vi "Autonomous Independent.vi"   [LabVIEW 2019]
doc: "This VI is called when autonomous begins, and will automatically be terminated when autonomous ends. You can carry out timed or sensor driven robot movement independently without needing to return to the caller."
uses:
  <vilib>/Rock Robotics/WPI/DriverStation/WPI_DriverStationDerivedRobotMode.ctl
  <vilib>/Rock Robotics/Network Tables/NT Read String.vi
  <vilib>/Rock Robotics/WPI/Utilities/WPI_GetSetVariantRefNum.vi
  <vilib>/Rock Robotics/Network Tables/NT Write Boolean.vi
  <vilib>/Rock Robotics/Network Tables/NT Write Number.vi
  <vilib>/Rock Robotics/Network Tables/NT Read Number.vi
  Robot Global Data.vi
  <vilib>/Rock Robotics/Network Tables/NT Write Numeric Array.vi
panel:
  # "Be sure to right-click and choose Data Operations>>Make Current Value default if you want to save the array values with the VI"
types:
  T1 = typedef "WPI_JoystickDevRef.ctl" = cluster{"Device":T2}
  T2 = typedef "WPI_JoystickDeviceEnum.ctl" = enum16{"USB 0", "USB 1", "USB 2", "USB 3", "USB 4", "USB 5"}
  T3 = typedef "WPI_MotorControlDeviceRef.ctl" = cluster{"DeviceStatus":errorcluster, "Type":T4, "PWM":cluster{"PWM Channel":T5, "DeadBand":T6}, "CAN":cluster{"Device Number":u8, "SetOutput VI Ref":variant, "GetOutput VI Ref":variant, "Enable VI Ref":variant, "Disable VI Ref":variant, "Data":variant}, "Invert":bool, "DIO PWM":cluster{"PWM \"Enable\" Channel":T5, "DIOChannel":T7, "PWM Rate":dbl}}
  T4 = typedef "WPI_MotorControlType.ctl" = enum16{"PWM", "CAN", "DIO PWM"}
  T5 = typedef "FPGA_DIOPWMChannel.ctl" = enum8{"PWM 0", "PWM 1", "PWM 2", "PWM 3", "PWM 4", "PWM 5", "PWM 6", "PWM 7", "PWM 8", "PWM 9", "PWM MXP 0", "PWM MXP 1", "PWM MXP 2", "PWM MXP 3", "PWM MXP 4", "PWM MXP 5", "PWM MXP 6", "PWM MXP 7", "PWM MXP 8", "PWM MXP 9", "Invalid"}
  T6 = typedef "WPI_PWMDeadband.ctl" = cluster{"Name":string, "maxPositivePwm":i32, "minPositivePwm":i32, "centerPwm":i32, "maxNegativePwm":i32, "minNegativePwm":i32, "angularRange":u16}
  T7 = typedef "FPGA_DIOChannel.ctl" = enum8{"DIO 0", "DIO 1", "DIO 2", "DIO 3", "DIO 4", "DIO 5", "DIO 6", "DIO 7", "DIO 8", "DIO 9", "DIO MXP 0", "DIO MXP 1", "DIO MXP 2", "DIO MXP 3", "DIO MXP 4", "DIO MXP 5", "DIO MXP 6", "DIO MXP 7", "DIO MXP 8", "DIO MXP 9", "DIO MXP 10", "DIO MXP 11", "DIO MXP 12", "DIO MXP 13", "DIO MXP 14", "DIO MXP 15", "SPI Port CS1", "SPI Port CS2", "SPI Port CS3", "SPI Port MISO", "SPI Port MOSI", "Invalid"}
  T8 = typedef "WPI_RobotDriveDevRef.ctl" = cluster{"DevStatus":errorcluster, "Motors[]":T3[], "Square Inputs":bool, "Max Output":dbl}
  T9 = typedef "WPI_DriverStationDerivedRobotMode.ctl" = enum16{"Init", "Execute", "Stop"}
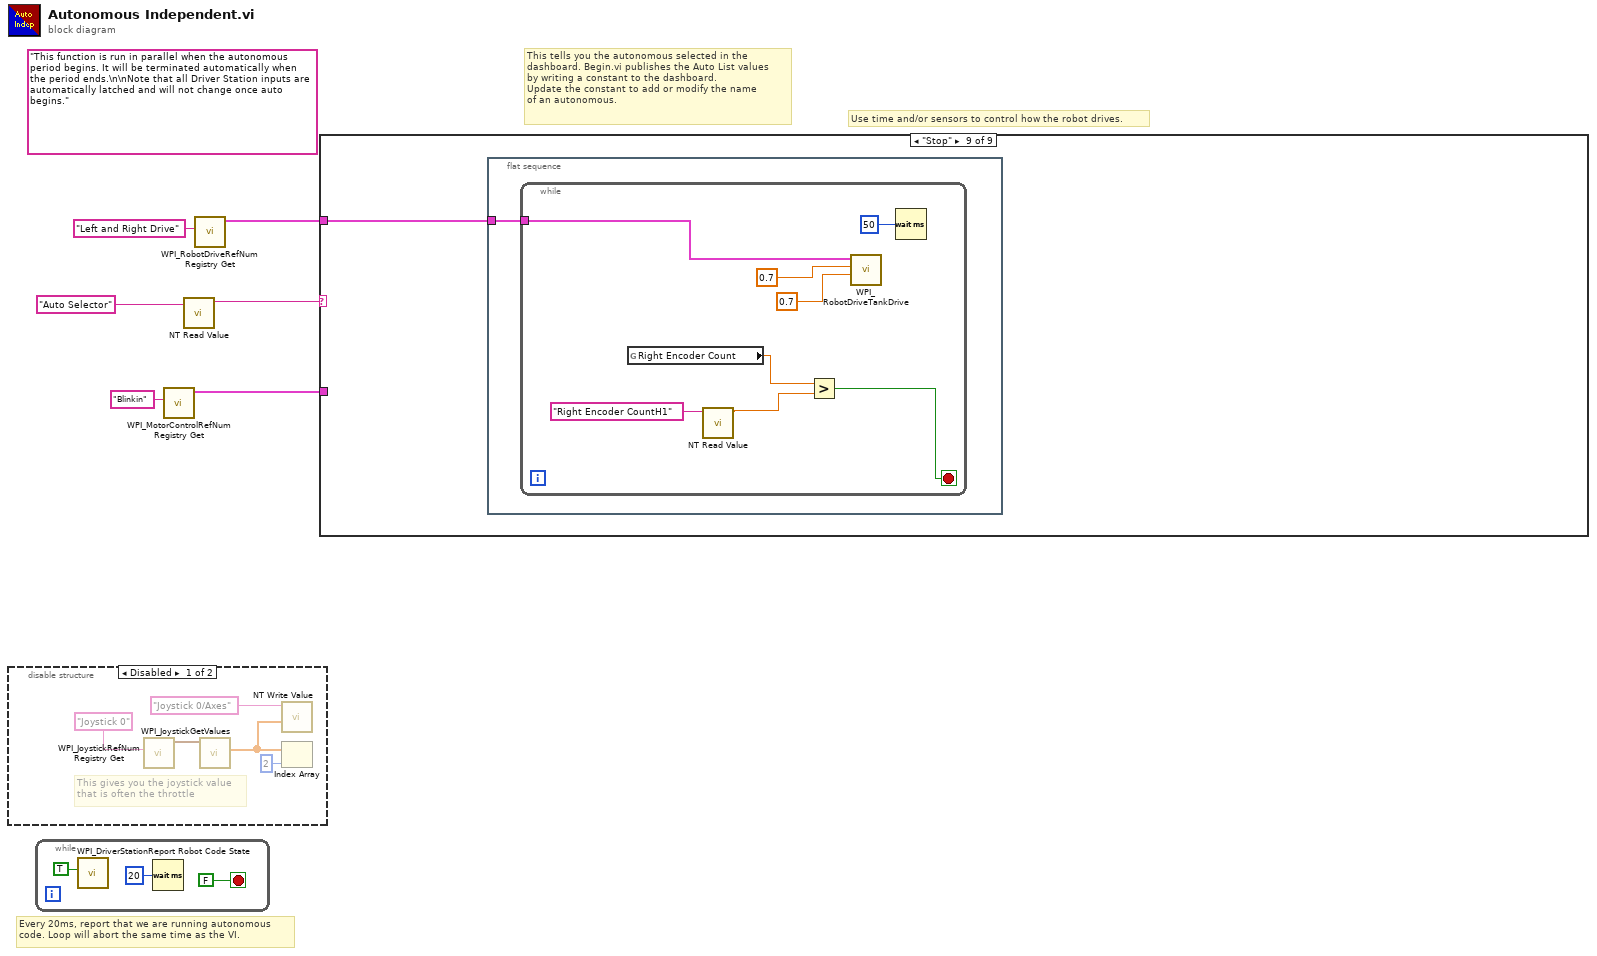
[diagram p0: block diagram]
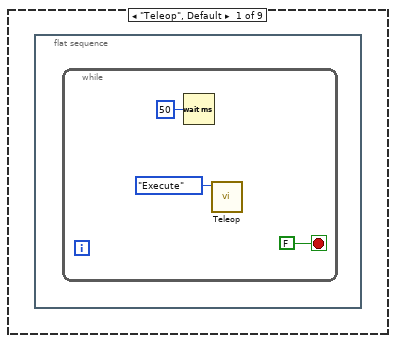
[diagram p3: hidden frame]
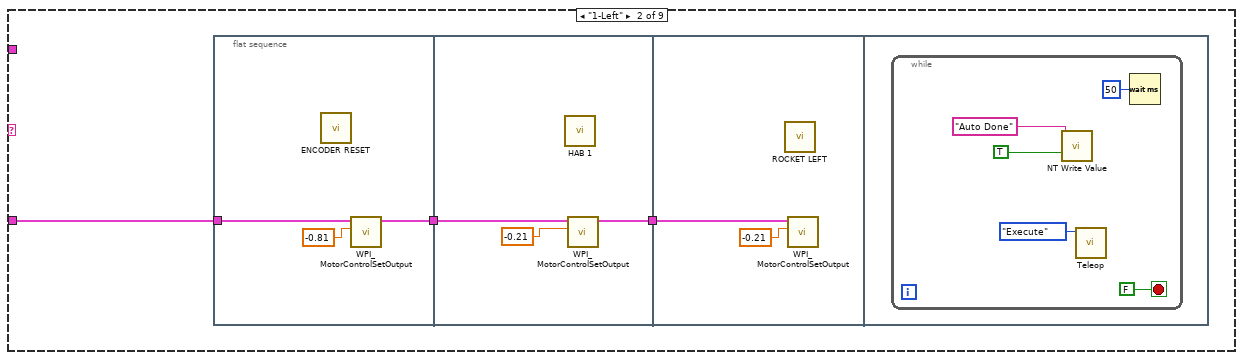
[diagram p4: hidden frame]
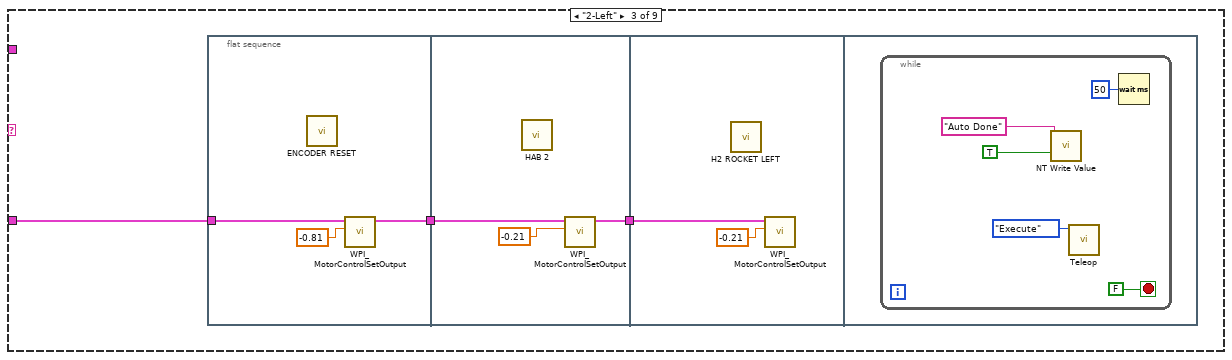
[diagram p5: hidden frame]
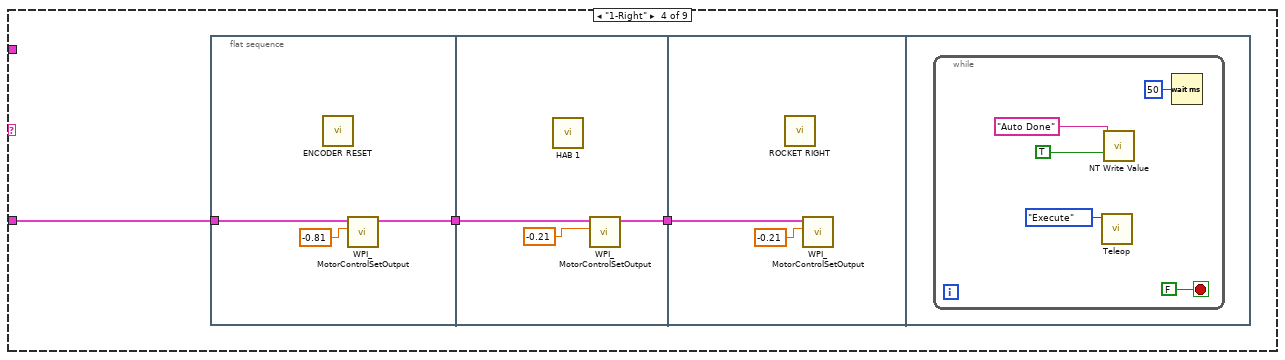
[diagram p6: hidden frame]
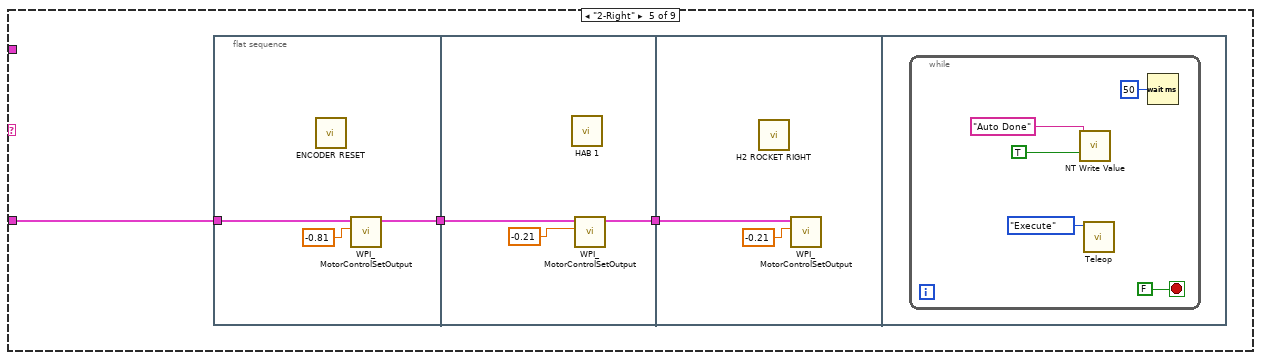
[diagram p7: hidden frame]
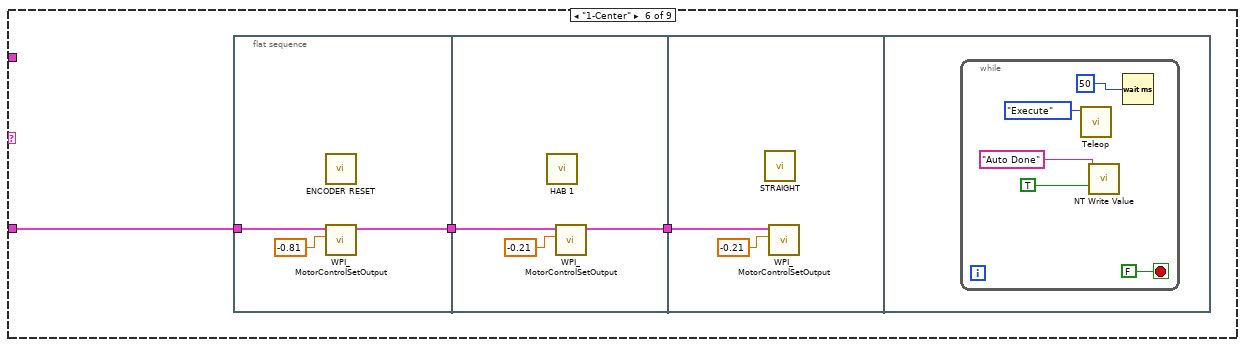
[diagram p8: hidden frame]
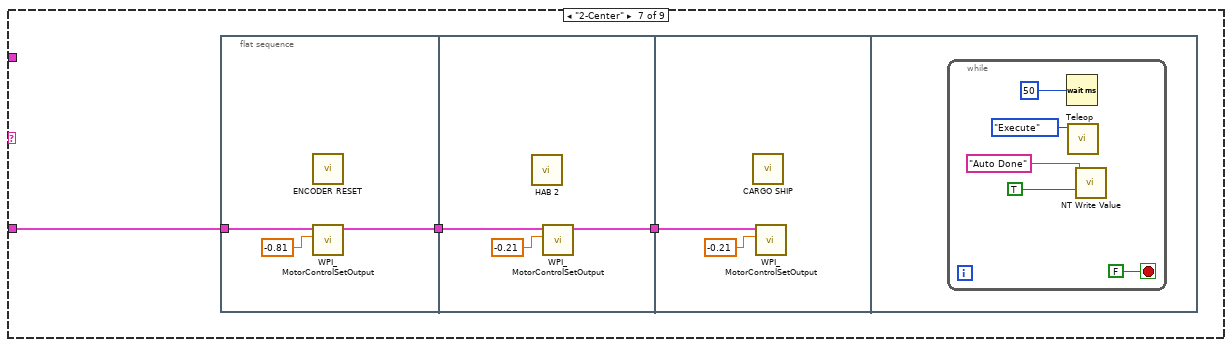
[diagram p9: hidden frame]
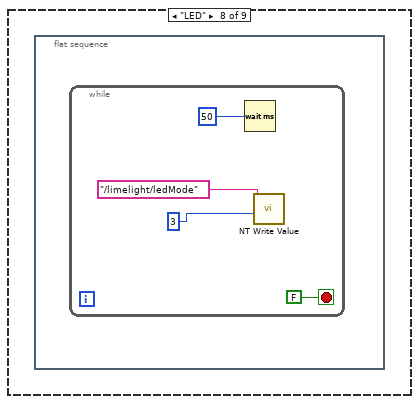
[diagram p10: hidden frame]
diagram:
  (unwired) "This function is run in parallel when the autonomous period begins. It will be terminated automatically when the period ends.\n\nNote that all Driver Station inputs are automatically latched and will not change once auto begins."
  # "This tells you the autonomous selected in the \ndashboard. Begin.vi publishes the Auto List values\nby writing a constant to the dashboard.\nUpdate the constant to add or modify the name\nof an autonomous."
  # "Every 20ms, report that we are running autonomous\ncode. Loop will abort the same time as the VI."
  # "Use time and/or sensors to control how the robot drives."
  n1 = disable-structure shown="Disabled" {
    frame Disabled {
      # "This gives you the joystick value\nthat is often the throttle"
      n2 = call <vilib>:"WPI_JoystickRefNum Registry Get.vi"("refnum name"="Joystick 0") -> ("JoystickDevRef"=w10:T1)  [unwired: 1 in, 9 out]
      n3 = call <vilib>:"WPI_JoystickGetValues.vi"("JoystickDevRef"=w10) -> ("Axes"=w8:dbl[])  [unwired: 6 in, 4 out]
      n4 = call-poly <vilib>:"NT Write Value.vi"("Numeric Array"=w8, "Name"="Joystick 0/Axes") -> ()  [unwired: 9 in, 1 out]
      n5 = Index Array(array=w8, index=2) -> ()  [unwired: 1 out]
    }
    frame Enabled {
    }
  }
  n6 = while {
    stop <- FALSE stop-if-true
    n7 = call <vilib>:"WPI_DriverStationReport Robot Code State.vi"("Autonomous"=TRUE) -> ()  [unwired: 10 in, 1 out]
    n8 = Wait (ms)(milliseconds to wait=u32 20) -> ()  [unwired: 1 out]
  }
  n9 = call <vilib>:"WPI_MotorControlRefNum Registry Get.vi"("refnum name"="Blinkin") -> ("MotorControlDevRef"=w5:T3)  [unwired: 9 in, 1 out]
  n10 = call-poly <vilib>:"NT Read Value.vi"("Name"="Auto Selector") -> ("String"=w3:string)  [unwired: 9 in, 1 out]
  n11 = call <vilib>:"WPI_RobotDriveRefNum Registry Get.vi"("refnum name"="Left and Right Drive") -> ("RobotDriveDevRef"=w1:T8)  [unwired: 9 in, 1 out]
  n12 = case shown="\"Stop\"" w3 {
    tunnel: w5 -> [_ w20 w36 w52 w68 w84 w100 _ _]
    tunnel: w1 -> [_ _ _ _ _ _ _ _ w118]
    frame "Teleop", Default {
      n13 = flat-sequence {
        frame #0 {
          n14 = while {
            stop <- FALSE stop-if-true
            n15 = Wait (ms)(milliseconds to wait=u32 50) -> ()  [unwired: 1 out]
            n16 = call "Teleop.vi"("Call Context"=WPI_DriverStationDerivedRobotMode."Execute") -> ()  [unwired: 11 in]
          }
        }
      }
    }
    frame "1-Left" {
      n17 = flat-sequence {
        tunnel: w20 -> [w23]
        tunnel: [w21] -> w19
        tunnel: w19 -> [w25]
        tunnel: [w24] -> w18
        tunnel: w18 -> [w27]
        frame #0 {
          n18 = call "ENCODER RESET.vi"() -> ()  [unwired: 12 in]
          n19 = call <vilib>:"WPI_MotorControlSetOutput.vi"("Output"=-0.81, "MotorControlDevRef"=w23) -> ("MotorControlDevRef"=w21:T3)  [unwired: 7 in, 2 out]
        }
        frame #1 {
          n20 = call "HAB 1.vi"() -> ()  [unwired: 12 in]
          n21 = call <vilib>:"WPI_MotorControlSetOutput.vi"("Output"=-0.21, "MotorControlDevRef"=w25) -> ("MotorControlDevRef"=w24:T3)  [unwired: 7 in, 2 out]
        }
        frame #2 {
          n22 = call "ROCKET LEFT.vi"() -> ()  [unwired: 12 in]
          n23 = call <vilib>:"WPI_MotorControlSetOutput.vi"("Output"=-0.21, "MotorControlDevRef"=w27) -> ()  [unwired: 7 in, 3 out]
        }
        frame #3 {
          n24 = while {
            stop <- FALSE stop-if-true
            n25 = call-poly <vilib>:"NT Write Value.vi"("Boolean"=TRUE, "Name"="Auto Done") -> ()  [unwired: 9 in, 1 out]
            n26 = call "Teleop.vi"("Call Context"=WPI_DriverStationDerivedRobotMode."Execute") -> ()  [unwired: 11 in]
            n27 = Wait (ms)(milliseconds to wait=u32 50) -> ()  [unwired: 1 out]
          }
        }
      }
    }
    frame "2-Left" {
      n28 = flat-sequence {
        tunnel: w36 -> [w39]
        tunnel: [w37] -> w35
        tunnel: w35 -> [w41]
        tunnel: [w40] -> w34
        tunnel: w34 -> [w43]
        frame #0 {
          n29 = call "ENCODER RESET.vi"() -> ()  [unwired: 12 in]
          n30 = call <vilib>:"WPI_MotorControlSetOutput.vi"("Output"=-0.81, "MotorControlDevRef"=w39) -> ("MotorControlDevRef"=w37:T3)  [unwired: 7 in, 2 out]
        }
        frame #1 {
          n31 = call "HAB 2.vi"() -> ()  [unwired: 12 in]
          n32 = call <vilib>:"WPI_MotorControlSetOutput.vi"("Output"=-0.21, "MotorControlDevRef"=w41) -> ("MotorControlDevRef"=w40:T3)  [unwired: 7 in, 2 out]
        }
        frame #2 {
          n33 = call "H2 ROCKET LEFT.vi"() -> ()  [unwired: 12 in]
          n34 = call <vilib>:"WPI_MotorControlSetOutput.vi"("Output"=-0.21, "MotorControlDevRef"=w43) -> ()  [unwired: 7 in, 3 out]
        }
        frame #3 {
          n35 = while {
            stop <- FALSE stop-if-true
            n36 = call-poly <vilib>:"NT Write Value.vi"("Boolean"=TRUE, "Name"="Auto Done") -> ()  [unwired: 9 in, 1 out]
            n37 = call "Teleop.vi"("Call Context"=WPI_DriverStationDerivedRobotMode."Execute") -> ()  [unwired: 11 in]
            n38 = Wait (ms)(milliseconds to wait=u32 50) -> ()  [unwired: 1 out]
          }
        }
      }
    }
    frame "1-Right" {
      n39 = flat-sequence {
        tunnel: w52 -> [w55]
        tunnel: [w53] -> w51
        tunnel: w51 -> [w57]
        tunnel: [w56] -> w50
        tunnel: w50 -> [w59]
        frame #0 {
          n40 = call "ENCODER RESET.vi"() -> ()  [unwired: 12 in]
          n41 = call <vilib>:"WPI_MotorControlSetOutput.vi"("Output"=-0.81, "MotorControlDevRef"=w55) -> ("MotorControlDevRef"=w53:T3)  [unwired: 7 in, 2 out]
        }
        frame #1 {
          n42 = call "HAB 1.vi"() -> ()  [unwired: 12 in]
          n43 = call <vilib>:"WPI_MotorControlSetOutput.vi"("Output"=-0.21, "MotorControlDevRef"=w57) -> ("MotorControlDevRef"=w56:T3)  [unwired: 7 in, 2 out]
        }
        frame #2 {
          n44 = call "ROCKET RIGHT.vi"() -> ()  [unwired: 12 in]
          n45 = call <vilib>:"WPI_MotorControlSetOutput.vi"("Output"=-0.21, "MotorControlDevRef"=w59) -> ()  [unwired: 7 in, 3 out]
        }
        frame #3 {
          n46 = while {
            stop <- FALSE stop-if-true
            n47 = call "Teleop.vi"("Call Context"=WPI_DriverStationDerivedRobotMode."Execute") -> ()  [unwired: 11 in]
            n48 = call-poly <vilib>:"NT Write Value.vi"("Boolean"=TRUE, "Name"="Auto Done") -> ()  [unwired: 9 in, 1 out]
            n49 = Wait (ms)(milliseconds to wait=u32 50) -> ()  [unwired: 1 out]
          }
        }
      }
    }
    frame "2-Right" {
      n50 = flat-sequence {
        tunnel: w68 -> [w71]
        tunnel: [w69] -> w67
        tunnel: w67 -> [w73]
        tunnel: [w72] -> w66
        tunnel: w66 -> [w75]
        frame #0 {
          n51 = call "ENCODER RESET.vi"() -> ()  [unwired: 12 in]
          n52 = call <vilib>:"WPI_MotorControlSetOutput.vi"("Output"=-0.81, "MotorControlDevRef"=w71) -> ("MotorControlDevRef"=w69:T3)  [unwired: 7 in, 2 out]
        }
        frame #1 {
          n53 = call "HAB 1.vi"() -> ()  [unwired: 12 in]
          n54 = call <vilib>:"WPI_MotorControlSetOutput.vi"("Output"=-0.21, "MotorControlDevRef"=w73) -> ("MotorControlDevRef"=w72:T3)  [unwired: 7 in, 2 out]
        }
        frame #2 {
          n55 = call "H2 ROCKET RIGHT.vi"() -> ()  [unwired: 12 in]
          n56 = call <vilib>:"WPI_MotorControlSetOutput.vi"("Output"=-0.21, "MotorControlDevRef"=w75) -> ()  [unwired: 7 in, 3 out]
        }
        frame #3 {
          n57 = while {
            stop <- FALSE stop-if-true
            n58 = call-poly <vilib>:"NT Write Value.vi"("Boolean"=TRUE, "Name"="Auto Done") -> ()  [unwired: 9 in, 1 out]
            n59 = call "Teleop.vi"("Call Context"=WPI_DriverStationDerivedRobotMode."Execute") -> ()  [unwired: 11 in]
            n60 = Wait (ms)(milliseconds to wait=u32 50) -> ()  [unwired: 1 out]
          }
        }
      }
    }
    frame "1-Center" {
      n61 = flat-sequence {
        tunnel: w84 -> [w87]
        tunnel: [w85] -> w83
        tunnel: w83 -> [w89]
        tunnel: [w88] -> w82
        tunnel: w82 -> [w91]
        frame #0 {
          n62 = call "ENCODER RESET.vi"() -> ()  [unwired: 12 in]
          n63 = call <vilib>:"WPI_MotorControlSetOutput.vi"("Output"=-0.81, "MotorControlDevRef"=w87) -> ("MotorControlDevRef"=w85:T3)  [unwired: 7 in, 2 out]
        }
        frame #1 {
          n64 = call "HAB 1.vi"() -> ()  [unwired: 12 in]
          n65 = call <vilib>:"WPI_MotorControlSetOutput.vi"("Output"=-0.21, "MotorControlDevRef"=w89) -> ("MotorControlDevRef"=w88:T3)  [unwired: 7 in, 2 out]
        }
        frame #2 {
          n66 = call "STRAIGHT.vi"() -> ()  [unwired: 12 in]
          n67 = call <vilib>:"WPI_MotorControlSetOutput.vi"("Output"=-0.21, "MotorControlDevRef"=w91) -> ()  [unwired: 7 in, 3 out]
        }
        frame #3 {
          n68 = while {
            stop <- FALSE stop-if-true
            n69 = call "Teleop.vi"("Call Context"=WPI_DriverStationDerivedRobotMode."Execute") -> ()  [unwired: 11 in]
            n70 = call-poly <vilib>:"NT Write Value.vi"("Boolean"=TRUE, "Name"="Auto Done") -> ()  [unwired: 9 in, 1 out]
            n71 = Wait (ms)(milliseconds to wait=50) -> ()  [unwired: 1 out]
          }
        }
      }
    }
    frame "2-Center" {
      n72 = flat-sequence {
        tunnel: w100 -> [w103]
        tunnel: [w101] -> w99
        tunnel: w99 -> [w105]
        tunnel: [w104] -> w98
        tunnel: w98 -> [w107]
        frame #0 {
          n73 = call "ENCODER RESET.vi"() -> ()  [unwired: 12 in]
          n74 = call <vilib>:"WPI_MotorControlSetOutput.vi"("Output"=-0.81, "MotorControlDevRef"=w103) -> ("MotorControlDevRef"=w101:T3)  [unwired: 7 in, 2 out]
        }
        frame #1 {
          n75 = call "HAB 2.vi"() -> ()  [unwired: 12 in]
          n76 = call <vilib>:"WPI_MotorControlSetOutput.vi"("Output"=-0.21, "MotorControlDevRef"=w105) -> ("MotorControlDevRef"=w104:T3)  [unwired: 7 in, 2 out]
        }
        frame #2 {
          n77 = call "CARGO SHIP.vi"() -> ()  [unwired: 12 in]
          n78 = call <vilib>:"WPI_MotorControlSetOutput.vi"("Output"=-0.21, "MotorControlDevRef"=w107) -> ()  [unwired: 7 in, 3 out]
        }
        frame #3 {
          n79 = while {
            stop <- FALSE stop-if-true
            n80 = Wait (ms)(milliseconds to wait=50) -> ()  [unwired: 1 out]
            n81 = call "Teleop.vi"("Call Context"=WPI_DriverStationDerivedRobotMode."Execute") -> ()  [unwired: 11 in]
            n82 = call-poly <vilib>:"NT Write Value.vi"("Boolean"=TRUE, "Name"="Auto Done") -> ()  [unwired: 9 in, 1 out]
          }
        }
      }
    }
    frame "LED" {
      n83 = flat-sequence {
        frame #0 {
          n84 = while {
            stop <- FALSE stop-if-true
            n85 = Wait (ms)(milliseconds to wait=50) -> ()  [unwired: 1 out]
            n86 = call-poly <vilib>:"NT Write Value.vi"("Numeric"=3, "Name"="/limelight/ledMode") -> ()  [unwired: 9 in, 1 out]
          }
        }
      }
    }
    frame "Stop" {
      n87 = flat-sequence {
        tunnel: w118 -> [w119]
        frame #0 {
          n88 = while {
            tunnel: w119 -> [w120]
            stop <- w123 stop-if-true
            n89 = global read "Robot Global Data.vi" "Right Encoder Count"() -> (w124:dbl)
            n90 = call-poly <vilib>:"NT Read Value.vi"("Name"="Right Encoder CountH1") -> ("Numeric"=w121:dbl)  [unwired: 9 in, 1 out]
            n91 = Greater?(x=w124, y=w121) -> (0:w123:bool)
            n92 = call <vilib>:"WPI_RobotDriveTankDrive.vi"("Right axis value"=0.7 ("Y axis value"), "Left axis value"=0.7 ("X axis value"), "RobotDriveDevRef"=w120) -> ()  [unwired: 6 in, 3 out]
            n93 = Wait (ms)(milliseconds to wait=u32 50) -> ()  [unwired: 1 out]
          }
        }
      }
    }
  }
